vi "Write Coords.vi"(6 "Coordinates":T1, 11 "Handle Drag Starting Msg in":refnum<class "Handle Drag Starting Msg.lvclass">) -> (3 "Handle Drag Starting Msg out":refnum<class "Handle Drag Starting Msg.lvclass">)   [LabVIEW 2020, in "File Explorer.lvlib" / "Handle Drag Starting Msg.lvclass"]
uses:
  <vilib>/gpm_packages/@cs/file-explorer-extension/Source/File Explorer/File Explorer Messages/Handle Drag Starting Msg/Handle Drag Starting Msg.lvclass
  <vilib>/Utility/miscctls.llb/LVPoint32TypeDef.ctl
  <vilib>/gpm_packages/@cs/file-explorer-extension/Source/File Explorer/File Explorer Messages/Handle Drag Starting Msg/Handle Drag Starting Msg.lvclass/Handle Drag Starting Msg.ctl
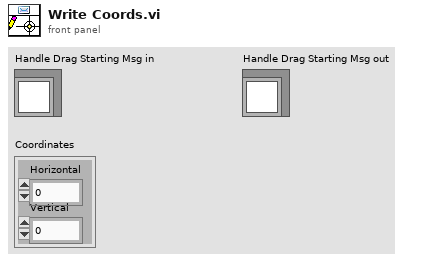
[diagram p1: front panel]
types:
  T1 = typedef "LVPoint32TypeDef.ctl" = cluster{"Horizontal":i32, "Vertical":i32}
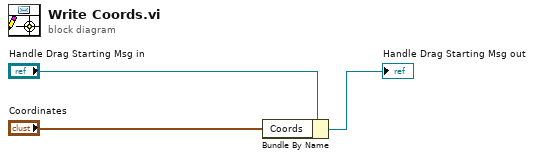
[diagram p0: block diagram]
diagram:
  n1 = Bundle By Name(cluster="Handle Drag Starting Msg in", "Coords"="Coordinates") -> (→"Handle Drag Starting Msg out":refnum<class "Handle Drag Starting Msg.lvclass">)
